vi "Write Instruments.vi"(8 "error in (no error)":errorcluster, 10 "Instruments":T1, 11 "Control Experiment out":refnum<class "Control Experiment.lvclass">) -> (0 "error out":errorcluster, 3 "Control Experiment out":refnum<class "Control Experiment.lvclass">)   [LabVIEW 2019, in "Control Experiment.lvclass"]
uses:
  Control Experiment.lvclass
  <userlib>/LevyLab/Krohn Hite 7008/Instrument.KH7008.lvclass
  <userlib>/LevyLab/Lockin-Multichannel/Instrument.Lockin/Instrument.Lockin.lvclass
  <userlib>/LevyLab/Instrument Framework/Instrument Types/Cryostat/Instrument.Cryostat.lvclass
  <userlib>/LevyLab/Instrument Framework/Instrument Types/CBridge/Instrument.CBridge.lvclass
  <userlib>/LevyLab/Instrument Framework/Instrument Types/Strain/Instrument.Strain.lvclass
  <userlib>/LevyLab/Instrument Framework/Instrument Types/VNA/Instrument.VNA.lvclass
  <userlib>/LevyLab/Instrument Framework/Instrument Types/VSource/Instrument.VSource.lvclass
  Typedefs/Instruments--cluster.ctl
  <userlib>/LevyLab/Instrument Framework/Instrument Types/Delay Line/Instrument.DelayLine.lvclass
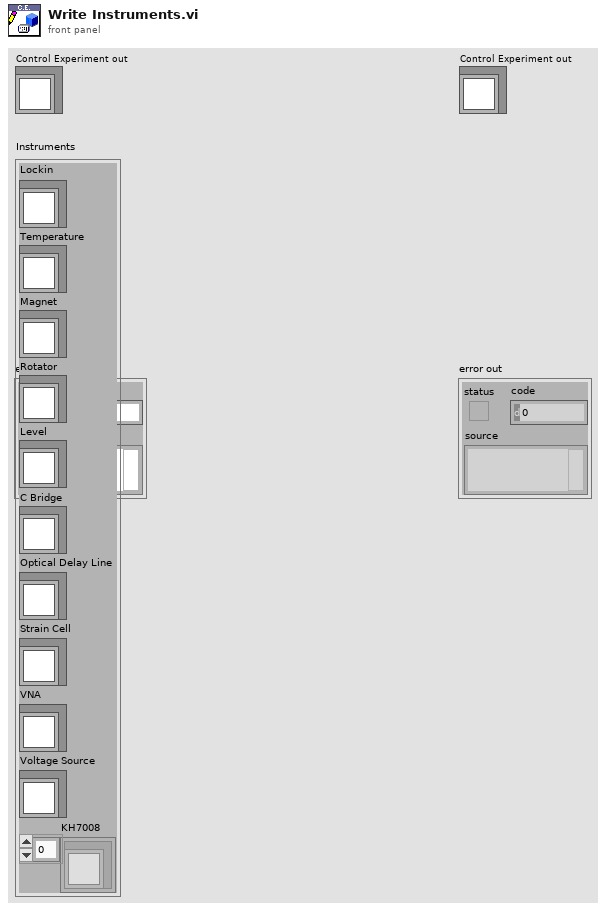
[diagram p1: front panel]
types:
  T1 = typedef "Control Experiment.lvclass/Instruments--cluster.ctl" = cluster{"Lockin":refnum<class "Instrument.Lockin.lvclass">, "Temperature":refnum<class "Instrument.Cryostat.lvclass">, "Magnet":refnum<class "Instrument.Cryostat.lvclass">, "Rotator":refnum<class "Instrument.Cryostat.lvclass">, "Level":refnum<class "Instrument.Cryostat.lvclass">, "C Bridge":refnum<class "Instrument.CBridge.lvclass">, "Optical Delay Line":refnum<class "Instrument.DelayLine.lvclass">, "Strain Cell":refnum<class "Instrument.Strain.lvclass">, "VNA":refnum<class "Instrument.VNA.lvclass">, "Voltage Source":refnum<class "Instrument.VSource.lvclass">, "KH7008":refnum<class "Instrument.KH7008.lvclass">[]}
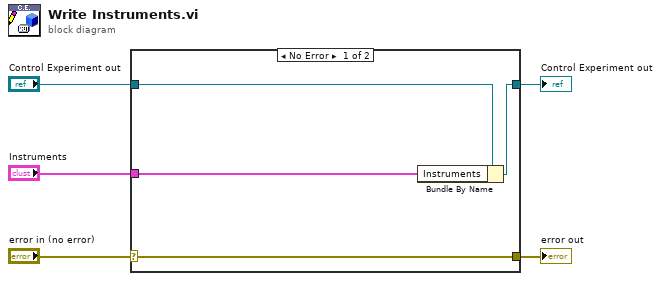
[diagram p0: block diagram]
diagram:
  n1 = case shown="No Error" "error in (no error)" {
    selector: "error in (no error)" -> [w9 w10]
    tunnel: [w9 w10] -> w4
    tunnel: [w7 w11] -> w2
    tunnel: "Control Experiment out" -> [w8 w11]
    tunnel: "Instruments" -> [w6 _]
    frame No Error {
      n2 = Bundle By Name(cluster=w8, "Instruments"=w6) -> (w7:refnum<class "Control Experiment.lvclass">)
    }
    frame Error {
    }
  }
  "error out" <- w4
  "Control Experiment out" <- w2
